vi "Autonomous Independent.vi"   [LabVIEW 2017]
doc: "This VI is called when autonomous begins, and will automatically be terminated when autonomous ends. You can carry out timed or sensor driven robot movement independently without needing to return to the caller."
uses:
  Robot Global Data.vi
panel:
  # "Be sure to right-click and choose Data Operations>>Make Current Value default if you want to save the array values with the VI"
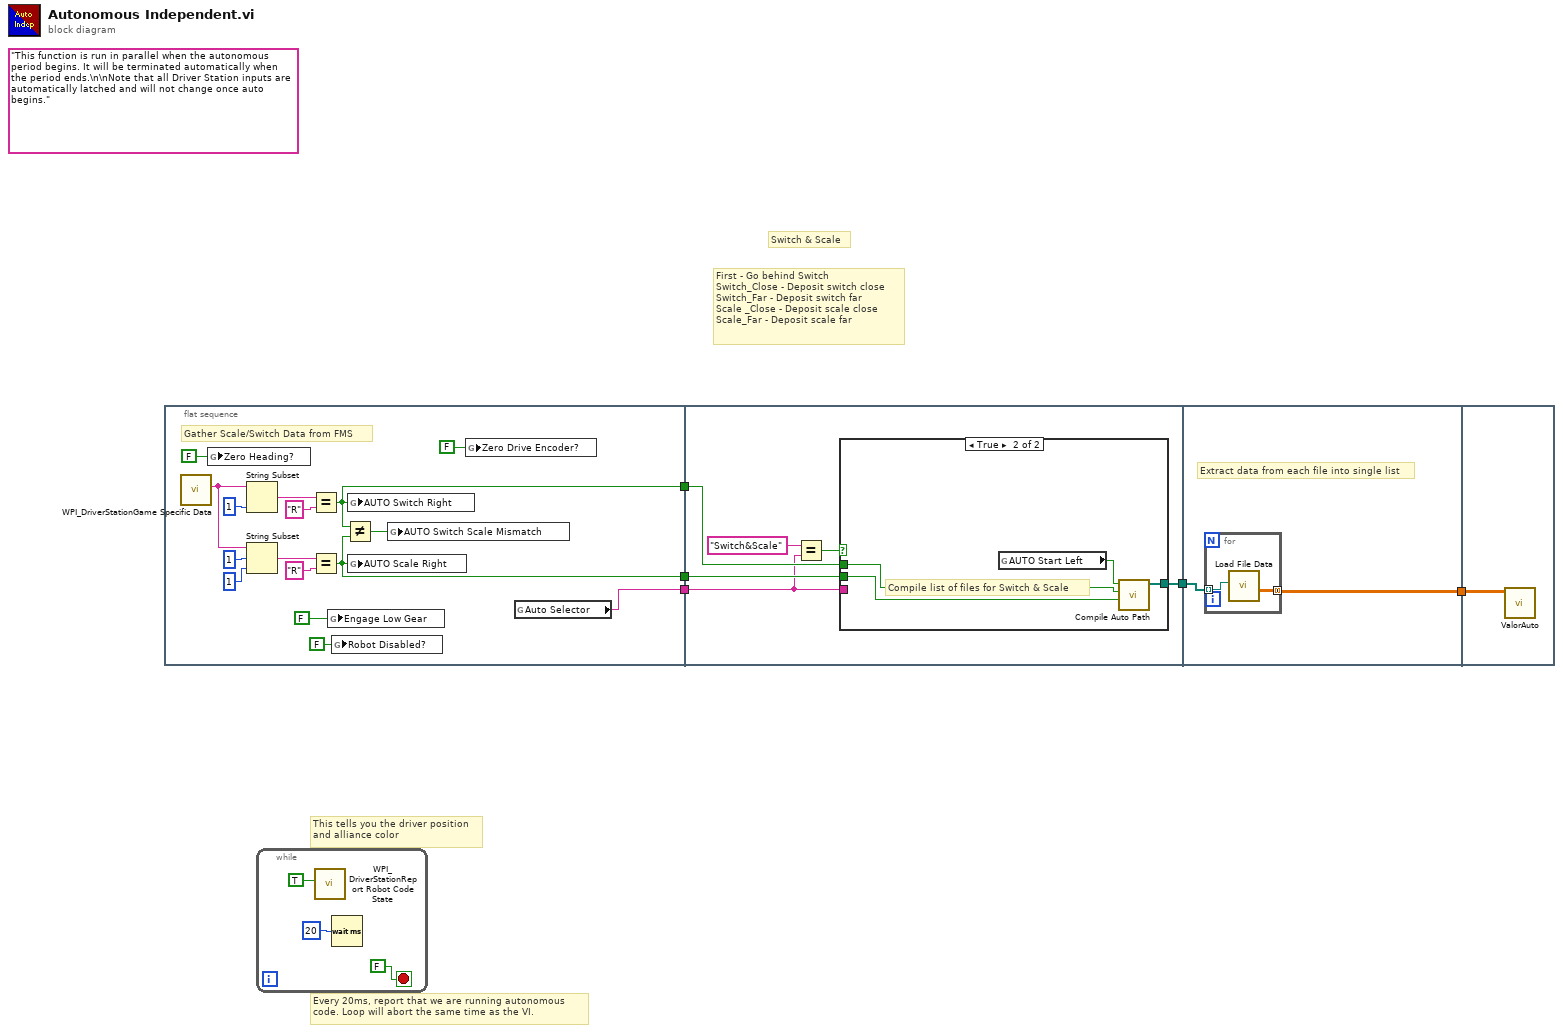
[diagram p0: block diagram]
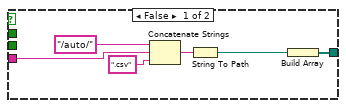
[diagram p2: hidden frame]
diagram:
  (unwired) "This function is run in parallel when the autonomous period begins. It will be terminated automatically when the period ends.\n\nNote that all Driver Station inputs are automatically latched and will not change once auto begins."
  # "Switch & Scale"
  # "First - Go behind Switch\nSwitch_Close - Deposit switch close\nSwitch_Far - Deposit switch far\nScale _Close - Deposit scale close\nScale_Far - Deposit scale far"
  # "Every 20ms, report that we are running autonomous\ncode. Loop will abort the same time as the VI."
  # "This tells you the driver position\nand alliance color"
  n1 = flat-sequence {
    tunnel: [w11] -> w5
    tunnel: [w10] -> w4
    tunnel: [w9] -> w1
    tunnel: w5 -> [w27]
    tunnel: w4 -> [w26]
    tunnel: [w25] -> w3
    tunnel: w1 -> [w22]
    tunnel: w3 -> [w39]
    tunnel: [w38] -> w2
    tunnel: w2 -> [w42]
    frame #0 {
      # "Gather Scale/Switch Data from FMS"
      n2 = call <vilib>:"WPI_DriverStationGame Specific Data.vi"() -> ("Game Specific Data"=w16:string)  [unwired: 11 in]
      n3 = global write "Robot Global Data.vi" "Zero Heading?"(FALSE ("Zero Heading?")) -> ()
      n4 = String Subset(string=w16, length (rest)=1 ("length (rest)")) -> (substring=w20:string)  [unwired: 1 in]
      n5 = String Subset(string=w16, offset (0)=1, length (rest)=1 ("length (rest)")) -> (substring=w18:string)
      n6 = Equal?(x=w20, y="R") -> (x = y?=w11:bool)
      n7 = Equal?(x=w18, y="R") -> (x = y?=w10:bool)
      n8 = global write "Robot Global Data.vi" "Engage Low Gear"(FALSE ("Zero Heading?")) -> ()
      n9 = global write "Robot Global Data.vi" "Robot Disabled?"(FALSE ("AUTO Start Left")) -> ()
      n10 = Not Equal?(x=w11, y=w10) -> (x != y?=w13:bool)
      n11 = global write "Robot Global Data.vi" "AUTO Switch Right"(w11) -> ()
      n12 = global write "Robot Global Data.vi" "AUTO Scale Right"(w10) -> ()
      n13 = global write "Robot Global Data.vi" "AUTO Switch Scale Mismatch"(w13) -> ()
      n14 = global write "Robot Global Data.vi" "Zero Drive Encoder?"(FALSE ("Zero Heading?")) -> ()
      n15 = global read "Robot Global Data.vi" "Auto Selector"() -> (w9:string)
    }
    frame #1 {
      n16 = Equal?(x="Switch&Scale", y=w22) -> (x = y?=w23:bool)
      n17 = case shown="True" w23 {
        tunnel: w27 -> [_ w36]
        tunnel: w26 -> [_ w35]
        tunnel: [w28 w34] -> w25
        tunnel: w22 -> [w33 _]
        frame False {
          n18 = Concatenate Strings("/auto/" ("string"), w33, ".csv" ("string")) -> (w30:string)
          n19 = String To Path(string=w30) -> (path=w29:path)
          n20 = Build Array(w29) -> (w28:path[])
        }
        frame True {
          # "Compile list of files for Switch & Scale"
          n21 = global read "Robot Global Data.vi" "AUTO Start Left"() -> (w37:bool)
          n22 = call "Compile Auto Path.vi"("Scale Right?"=w35, "Switch Right?"=w36, "Start Left?"=w37) -> ("Auto Paths"=w34:path[])  [unwired: 8 in]
        }
      }
    }
    frame #2 {
      # "Extract data from each file into single list"
      n23 = for {
        tunnel: w39 -> [w41] mode=indexing
        tunnel: [w40] -> w38 mode=concatenating
        n24 = call "Load File Data.vi"("Path"=w41) -> ("Auto Data"=w40:dbl[][])  [unwired: 10 in]
      }
    }
    frame #3 {
      n25 = call "ValorAuto.vi"("Steps"=w42) -> ()  [unwired: 11 in]
    }
  }
  n26 = while {
    stop <- FALSE stop-if-true
    n27 = call <vilib>:"WPI_DriverStationReport Robot Code State.vi"("Autonomous"=TRUE) -> ()  [unwired: 10 in, 1 out]
    n28 = Wait (ms)(milliseconds to wait=u32 20) -> ()  [unwired: 1 out]
  }
